vi "Sort 2 Column Array By First Column.vi"(11 "原始座標陣列":cluster{"X":dbl, "Y":dbl}[](array[cluster])=[{"X"=13.0, "Y"=100.0}, {"X"=12.0, "Y"=100.0}, {"X"=11.0, "Y"=100.0}, {"X"=22.0, "Y"=200.0}, {"X"=21.0, "Y"=200.0}, {"X"=24.0, "Y"=200.0}, {"X"=23.0, "Y"=200.0}, {"X"=33.0, "Y"=300.0}, {"X"=31.0, "Y"=300.0}, {"X"=34.0, "Y"=300.0}, {"X"=32.0, "Y"=300.0}, {"X"=35.0, "Y"=300.0}, {"X"=46.0, "Y"=400.0}, {"X"=44.0, "Y"=400.0}, {"X"=45.0, "Y"=400.0}, {"X"=43.0, "Y"=400.0}, {"X"=41.0, "Y"=400.0}, {"X"=42.0, "Y"=400.0}]) -> (3 "已完成排序座標陣列":cluster{"X":dbl, "Y":dbl}[][](array[cluster]))   [LabVIEW 2015]
panel:
  out "座標點數":i32
  out "輸入座標":dbl[][](array[numeric])
  in  "X個數":i32=5
  in  "Y個數":i32=5
  in  "分割閥值":dbl=75.0 format="%#_13g"
  in  "繪出結果?":bool=TRUE
  out "Image":T1(plugin-control)
  out "Array 2":errorcluster[](array[cluster])
  out "處理點數y":i32
  out "第一次排序結果之次要陣列":dbl[](array[numeric])
  out "第一次排序結果之主要陣列":dbl[](array[numeric])
  out "已完成排序陣列":dbl[][][](array[numeric])
  out "以各排數量切割之次要陣列":dbl[][](array[numeric])
  out "各排數量":i32[](array[numeric])
  out "以各排數量切割之主要陣列":dbl[][](array[numeric])
  out "第一次排序結果_X":dbl[](array[numeric])
  out "第一次排序結果_Y":dbl[](array[numeric])
  in  "主排序參考目標":enum16{"X排序", "Y排序"}(ring)
  out "第一次排序結果":dbl[][](array[numeric])
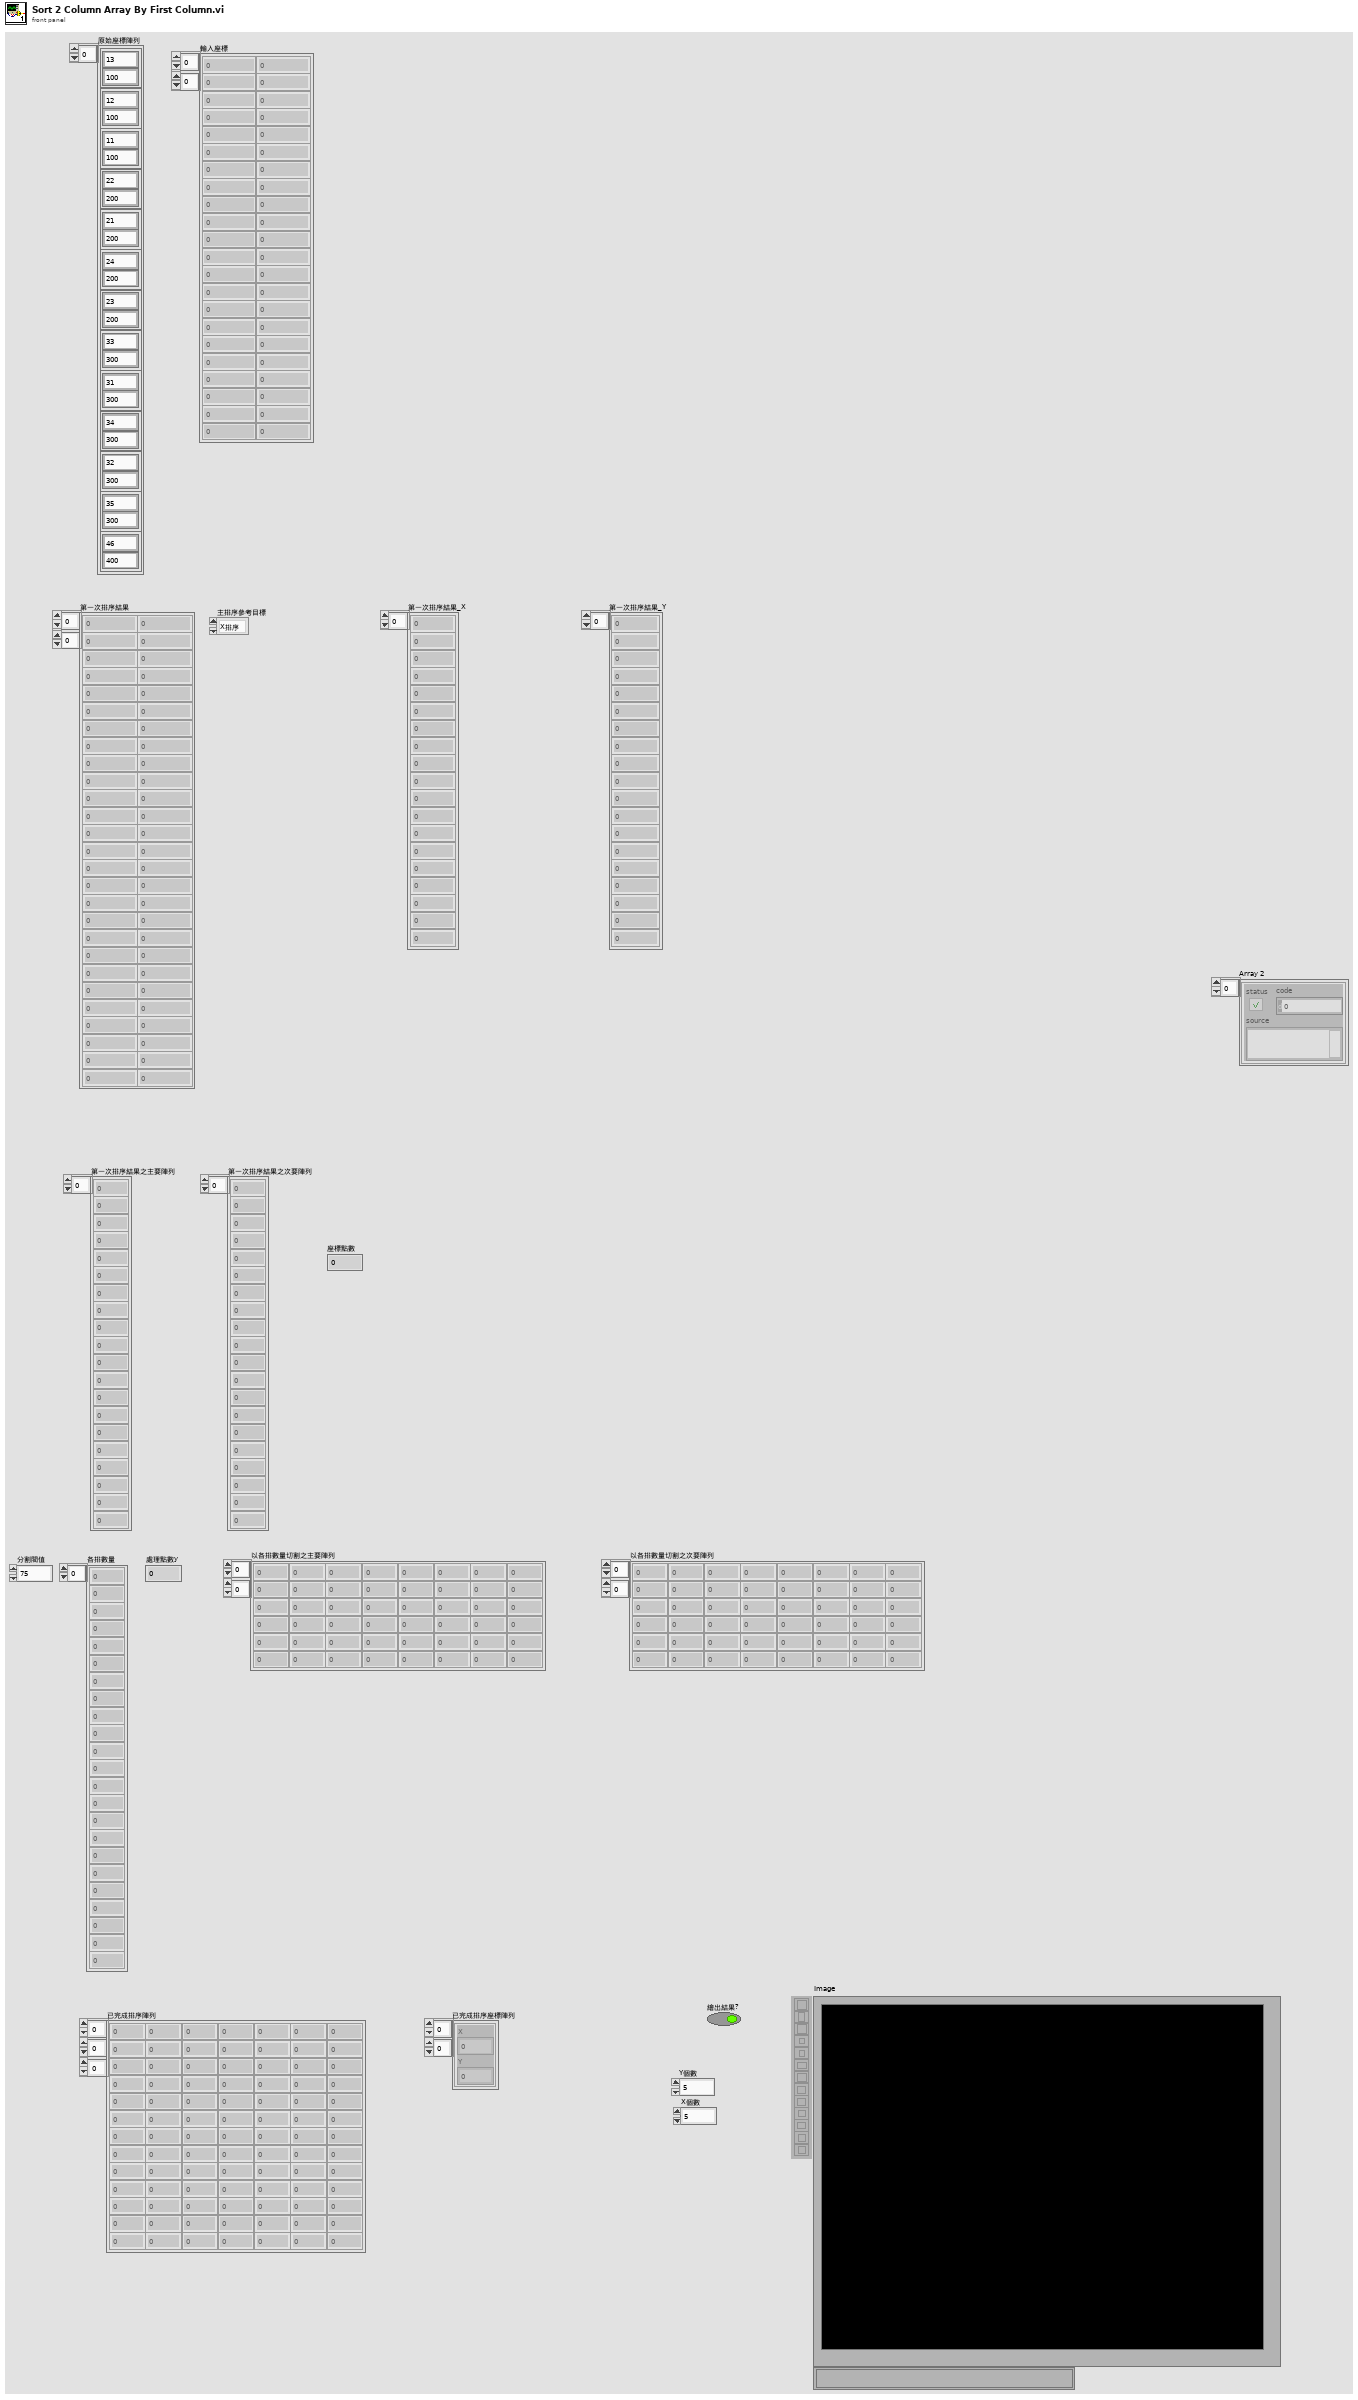
[diagram p1: front panel]
types:
  T1 = typedef "IMAQ Image.ctl" = refnum<image>
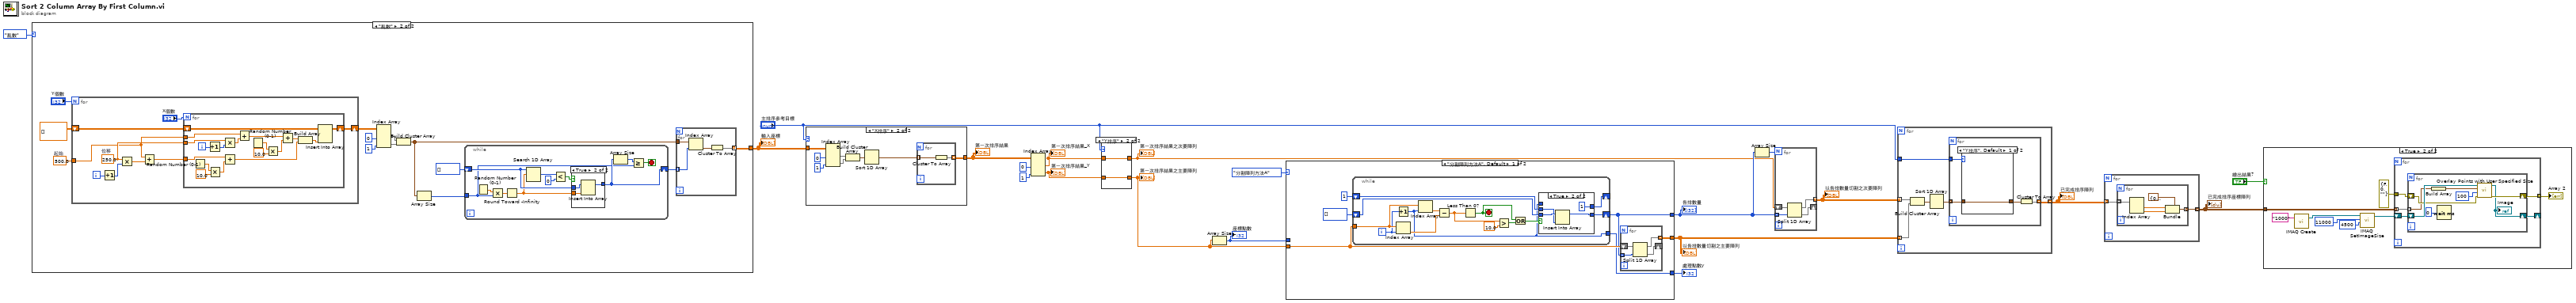
[diagram p0: block diagram]
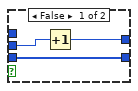
[diagram p2: hidden frame]
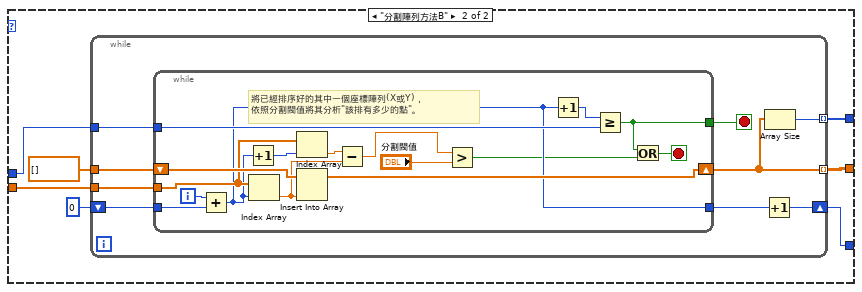
[diagram p3: hidden frame]
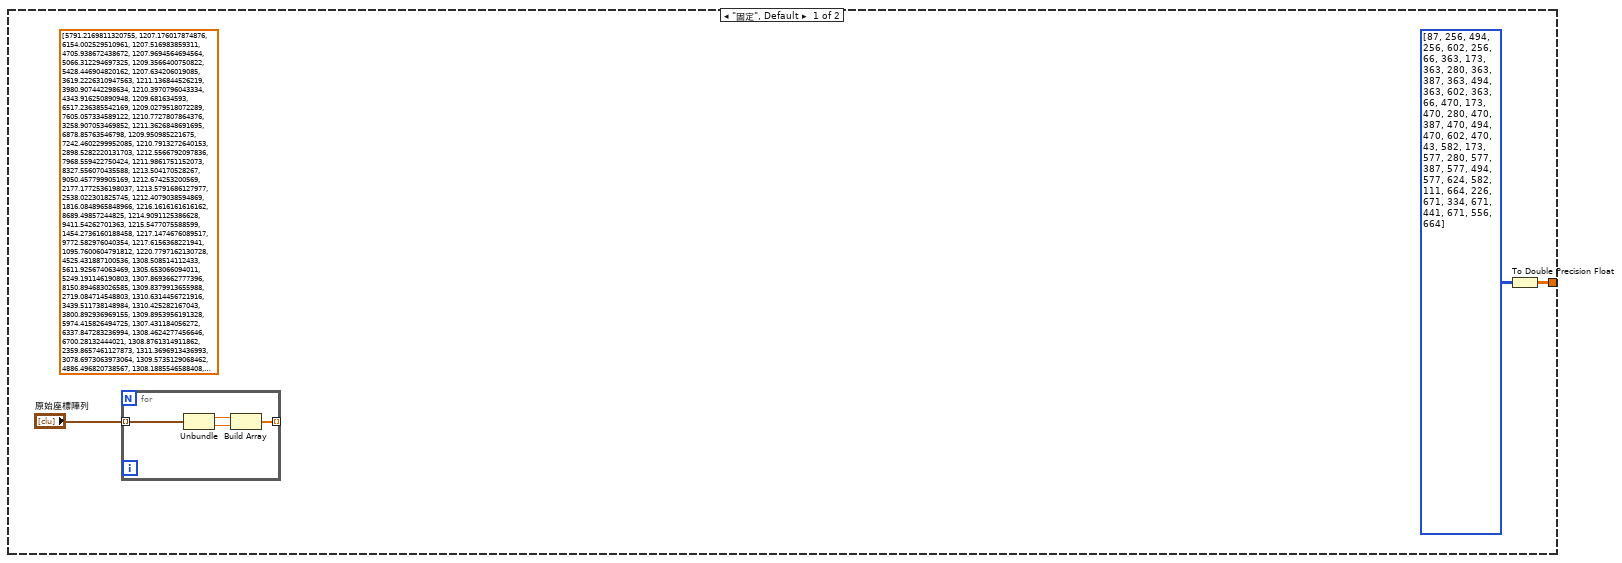
[diagram p4: hidden frame]
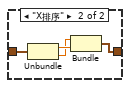
[diagram p7: hidden frame]
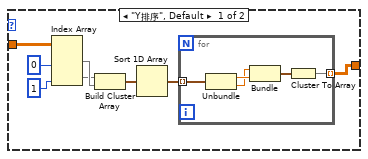
[diagram p9: hidden frame]
diagram:
  n1 = case shown="\"亂數\"" enum16{"固定", "亂數"}."亂數" {
    tunnel: [w21 w32] -> w6
    frame "固定", Default {
      (unwired) dbl[][] [[5791.2169811320755, 1207.176017874876], [6154.002529510961, 1207.516983859311], [4705.938672438672, 1207.9694564694564], [5066.312294697325, 1209.3566400750822], [5428.446904820162, 1207.634206019085], [3619.2226310947563, 1211.136844526219], [3980.907442298634, 1210.3970796043334], [4343.916250890948, 1209.681634593], [6517.236385542169, 1209.0279518072289], [7605.057334589122, 1210.7727807864376], [3258.907053469852, 1211.3626848691695], [6878.85763546798, 1209.950985221675], [7242.4602299952085, 1210.7913272640153], [2898.5282220131703, 1212.5566792097836], [7968.559422750424, 1211.9861751152073], [8327.556070435588, 1213.504170528267], [9050.457799905169, 1212.674253200569], [2177.1772536198037, 1213.5791686127977], [2538.022301825745, 1212.4079038594869], [1816.0848965848966, 1216.1616161616162], [8689.49857244825, 1214.9091125386628], [9411.54262701363, 1215.5477075588599], [1454.2736160188458, 1217.1474676089517], [9772.582976040354, 1217.6156368221941], [1095.7600604791812, 1220.7797162130728], [4525.431887100536, 1308.508514112433], [5611.925674063469, 1305.653066094011], [5249.191146190803, 1307.8693662777396], [8150.894683026585, 1309.8379913655988], [2719.084714548803, 1310.6314456721916], [3439.511738148984, 1310.425282167043], [3800.892936969155, 1309.8953956191328], [5974.415826494725, 1307.431184056272], [6337.847283236994, 1308.4624277456646], [6700.28132444021, 1308.8761314911862], [2359.8657461127873, 1311.3696913436993], [3078.6973063973064, 1309.5735129068462], [4886.496820738567, 1308.1885546588408], [7062.827751196172, 1309.4813397129187], [7427.45506669787, 1309.2068804118885], [8511.356658376668, 1311.258421885598], [8872.234061930783, 1311.655510018215], [4162.5688587086015, 1309.666428401239], [7788.041149425288, 1310.5857471264367], [1635.5710637352877, 1313.0397512769264], [1997.7501715069745, 1312.5035444774753], [9232.897453387903, 1313.3672123692588], [1274.6067873303168, 1317.8484162895927], [9593.201644660643, 1315.2645355570999], [9952.616504854368, 1317.176499875529], [5430.564612326044, 1403.6607852882703], [5793.774098695985, 1404.0516491945793], [6155.000251130085, 1403.7762430939226], [6518.11789807364, 1405.2377468910022], [4344.622950819672, 1406.5009643201543], [3619.45225714961, 1408.1621366107304], [7245.313248594475, 1408.0041554632119], [3258.734342012667, 1409.54890921886], [4707.38623046875, 1409.024169921875], [5068.421871049305, 1406.161567635904], [6882.053212358999, 1407.822216772928], [7608.443792155883, 1407.1306520109918], [2179.6376459143967, 1409.6850680933853], [3980.357344632768, 1409.775188323917], [7969.418336292163, 1407.645447628709], [8331.37233032748, 1408.6473659231135], [8692.269665567594, 1409.7538860103627], [2897.7616095307562, 1408.684172137126], [9053.6467124632, 1408.6459764474976], [2539.6725509696666, 1410.0730979612133], [1099.072462077013, 1414.2942823803967], [1817.3156834873253, 1413.0348258706467], [9414.970602828082, 1413.0022326966014], [9773.850379251284, 1414.3944213359432], [1455.220919100048, 1414.8228817616084], [5612.357605177994, 1502.180690399137], [4526.020811654526, 1502.9622788761706], [5247.853276353277, 1502.6335146335146], [5974.880021715527, 1502.6471226927254], [7788.572317880795, 1503.4405298013246], [8873.339039345938, 1505.144098109351], [6335.7773246329525, 1503.1606851549755], [4162.258917278016, 1506.8547938274728], [4886.88221614227, 1504.3124487004104], [6699.960096411355, 1503.6459560792716], [7065.031008783604, 1504.9840298110194], [7427.821718627194, 1505.8352108986114], [8150.256849315068, 1507.4307729941293], [8512.864804745428, 1508.1668314384578], [3800.291616477957, 1510.511443025777], [2359.2007088474666, 1507.0719348910475], [3077.414345769837, 1506.1037834997373], [3438.0564182194616, 1505.6392339544514], [9234.197371844914, 1507.5016913869372], [2716.955280172414, 1506.9234913793102], [1277.1903353057198, 1513.2260848126232], [1636.1105111591073, 1511.6306695464364], [1996.1912561258705, 1510.1307712148568], [9595.101593625497, 1512.0701195219124], [9952.666338305657, 1514.8809456797073], [6516.624943617501, 1607.9104645917907], [3616.434411500449, 1609.2830188679245], [3255.1358316452847, 1611.067521944632], [5066.782830573827, 1609.6119301428896], [6154.794930875576, 1608.5082949308755], [2895.820072743805, 1611.7272107297113], [4342.289616252821, 1610.3690744920993], [4705.4812142038945, 1610.4215349369988], [5427.558903488899, 1610.066606252832], [3978.4939475453934, 1610.3730105357542], [5790.527250608273, 1608.66399026764], [7242.933211344922, 1610.0388838060385], [7968.398886827458, 1610.7219387755101], [8691.733163028333, 1611.2183000464468], [9051.415883668904, 1612.092841163311], [6879.367298578199, 1610.8947867298577], [7605.550802779775, 1610.9796309609394], [9772.936148874527, 1614.2090483619345], [2537.1703652334722, 1613.1026352288488], [8329.660801564027, 1611.8164711632453], [9413.658141612686, 1613.2977440250168], [2174.5085707667363, 1615.4067639564512], [1454.8072275676884, 1620.3620496755427], [1098.2838932570885, 1618.710507505361], [1813.765814112811, 1619.6268554464489], [3432.7249308871574, 1714.0794169389294], [3795.35187044941, 1715.1995982927442], [4156.692948090108, 1716.0034280117532], [3073.052139379964, 1716.205995388163], [1632.0854131330263, 1718.6629512963411], [6330.915481832543, 1712.7777777777778], [8872.46767411301, 1717.6349540078843], [2714.7747580044675, 1716.6056093323405], [5969.166583229036, 1713.5344180225281], [6694.592108735814, 1714.9918184217472], [8508.792178917081, 1715.5417211613915], [1989.1021611001966, 1719.932956777996], [2353.5285641418004, 1719.878857434328], [5606.145459209852, 1716.39763981529], [7058.01411136537, 1715.0333079074499], [7421.791013584117, 1715.689132706374], [4519.88543328017, 1716.199893673578], [5243.284035133041, 1717.7452854559544], [7783.365578231293, 1717.2462585034014], [9232.259290072103, 1719.4728230726566], [1272.845079285175, 1720.5801661213188], [4882.937808219178, 1715.6323287671232], [8144.936657681941, 1717.1366576819407], [9591.000678426051, 1722.3915875169607], [9949.065279868619, 1723.254139865882], [4704.614984155726, 1811.9834766862834], [5786.604245164532, 1809.6865109269029], [6514.535163776493, 1813.2603564547205], [6877.67354965585, 1811.9594395280235], [6151.978198370867, 1813.089602299952], [3978.3221362977283, 1814.329386176897], [7240.83000997009, 1812.3277666999004], [7965.428588897041, 1815.9814135485449], [2534.981555834379, 1816.826850690088], [3615.618245699055, 1813.1737339471772], [4341.0246138996135, 1814.5381274131273], [5426.583291010666, 1811.312341289995], [8328.642644135189, 1815.0099403578529], [9052.143729743206, 1816.426576913488], [1815.0420583273078, 1819.9110629067245], [2895.753032928943, 1813.921020054469], [3253.824297438448, 1815.028848545138], [5065.478394303953, 1813.887061134299], [9414.352200457899, 1817.40422284406], [1098.6733201091, 1819.5578973468882], [2173.020701412567, 1819.3468095470043], [7603.653050672182, 1814.8753877973113], [1454.524729891957, 1821.038175270108], [8690.614173228347, 1814.9613681102362], [9773.988752556237, 1818.053680981595], [5247.1742229492875, 1908.279738256602], [5610.254849263847, 1908.1423229726572], [5972.489056087551, 1909.0362517099863], [6334.6076212471135, 1908.3951501154734], [7059.915295480881, 1908.824333719583], [7423.796435272045, 1910.078330206379], [7785.741147882434, 1910.896551724138], [4159.929595375723, 1910.3260115606936], [3437.6755601755603, 1913.949641949642], [4885.988111888112, 1910.7888111888112], [6696.816946348381, 1909.472465138265], [8148.402939804013, 1912.7727484834345], [2356.2925696594425, 1913.7811383662777], [2716.1378404204493, 1914.0993788819876], [3077.4003200731595, 1915.6213991769548], [3798.951251489869, 1912.8746126340882], [4523.41652344709, 1912.9629265897372], [9235.39332096475, 1913.7284322820037], [8509.45624256837, 1914.235196195006], [8873.527777777777, 1913.6053639846743], [9596.565009560229, 1914.8814531548758], [1636.0460588793921, 1919.2863247863247], [1996.2744091668656, 1918.7428980663642], [1279.4822637106183, 1920.5913652275378], [9952.766458852868, 1918.4258104738155], [6153.8170227429355, 2009.859637031932], [5066.484104721832, 2009.921458625526], [5789.492005643076, 2009.0002351281448], [5430.319796353303, 2008.9040966137816], [6517.169457067687, 2010.6376464960535], [6880.849392165691, 2012.3572714993247], [9055.709640745794, 2013.1377899045021], [3258.352574653186, 2014.5713613919586], [4705.719306466729, 2012.4835988753514], [7243.692893401016, 2011.9864636209813], [7607.454435288415, 2010.9663111972854], [7968.672670230072, 2012.3434812921219], [2897.9132035146044, 2014.5832343861316], [4343.976258649487, 2012.3120973514674], [8330.214816535068, 2013.349280074315], [3620.0517077798863, 2014.5493358633776], [3982.5302308974055, 2014.098309926208], [8693.775339002528, 2013.7924615031027], [2538.751615992339, 2015.047402441944], [9415.60828182942, 2015.435846724351], [2177.8562231759656, 2016.5591320934668], [9778.519986216403, 2018.1157822191592], [1817.681731909846, 2020.0873072360616], [1457.2464114832535, 2021.4196172248803], [1101.999758337361, 2022.1652972450458], [5248.732352237377, 2107.517827231395], [5973.682421227198, 2108.479270315091], [6700.691815856778, 2109.379446640316], [5612.669209105844, 2111.2762262379724], [7425.028975428836, 2110.2329624478443], [4887.984679665738, 2112.0299442896935], [6335.250118315192, 2111.0795078088026], [7788.795105566219, 2112.734404990403], [8150.576462459696, 2112.7206356517736], [8513.043503890593, 2111.8389530771046], [3801.8130515559683, 2113.5673478866697], [4525.211808809747, 2112.285613870665], [9235.167302192564, 2114.0865109628216], [2360.203281027104, 2115.401569186876], [2719.848698352042, 2113.9842369238117], [3079.9432965484857, 2113.6583705095095], [3440.210061884025, 2113.863167545267], [7062.920090239848, 2113.2161006886727], [4164.457772621809, 2114.2498839907194], [8875.46652922629, 2112.535774921174], [1998.6349448486271, 2115.715090354377], [9598.689484126984, 2117.3263888888887], [9954.744780152298, 2119.186809137804], [1639.7413207089098, 2120.402767662054], [1279.489117577478, 2121.8142890939203], [5431.053639360893, 2207.2916560994167], [6519.0869934481925, 2208.044892016501], [5792.554679802955, 2208.185960591133], [6154.561583577713, 2207.697458455523], [2899.03954050786, 2211.010882708585], [4707.999880753637, 2210.989983305509], [5068.351178781925, 2209.5230844793714], [6880.464836832785, 2209.094105742474], [7607.18498890806, 2209.4397337934433], [7969.78310727497, 2210.7551171393343], [3260.349441476445, 2212.7042253521126], [7244.3662109375, 2211.40087890625], [8331.217961405246, 2210.521276595745], [3623.0323997151672, 2213.4051744600047], [8694.145669291338, 2212.9379921259842], [3983.87895256917, 2211.9426877470355], [4344.828294280675, 2211.371126228269], [2540.2300098716682, 2214.078232971372], [9053.753157894736, 2212.271052631579], [2180.4587576374747, 2213.516547861507], [9414.56498194946, 2214.3120165033524], [1457.543881033642, 2217.4256460263286], [1820.8730694980695, 2219.265926640927], [9778.070615623383, 2216.237454733575], [1101.8869002284844, 2223.269611576542], [3441.5759493670885, 2307.637921940928], [5612.339923643305, 2305.1298063812383], [7062.993651204975, 2308.5752785695777], [4887.433227344992, 2306.98675145734], [5973.299479166667, 2306.385677083333], [6337.661087339542, 2308.794613642084], [4164.20913526701, 2307.685551640011], [4524.341320553781, 2305.896432374867], [5250.014176663031, 2305.5981461286806], [6700.81314699793, 2308.371376811594], [7425.287467362924, 2308.0046997389036], [7787.878064856314, 2308.0487740574745], [2719.438112429087, 2310.4272821041773], [3080.6123244929795, 2309.9682787311494], [3801.5416103755742, 2307.9921642799245], [8150.205319148936, 2309.8574468085108], [2362.5581613508443, 2310.08818011257], [8512.328911748782, 2308.986193827829], [2001.6717537506468, 2314.1324366270046], [8873.817425083242, 2310.0826859045505], [9234.317637452368, 2311.2874251497005], [9597.190749863164, 2313.4395183360703], [9954.403873140613, 2316.639489194499], [1639.6540974680097, 2315.3972229784918], [1279.6960380756368, 2320.3174684846927], [8330.202048007048, 2413.715481171548], [1096.627214902317, 2421.915720127215], [5793.369089316988, 2413.4614711033273], [6156.94052464948, 2411.7476255088195], [3981.7318511796734, 2415.4820780399273], [5068.8699074074075, 2412.4949074074075], [5431.829401290897, 2413.719563765858], [7243.78610919143, 2412.134761575674], [7605.668177697189, 2413.038984587489], [7967.357369975017, 2413.8964342493755], [4345.859130231471, 2413.3362169745146], [4707.703206141341, 2414.1840144502144], [6518.28573104905, 2412.7146209809903], [6880.357748469148, 2413.0977390485164], [3622.2240517828754, 2414.682262094027], [8691.513750592698, 2415.5320056899004], [2538.295429083576, 2417.556800358503], [2900.3592007434945, 2415.75906133829], [3261.9175365344468, 2416.071213175597], [9051.614809454897, 2415.5800771828267], [9412.444, 2418.5181176470587], [2180.4168634860653, 2419.272319319792], [9774.410749506904, 2419.995315581854], [1458.014869888476, 2422.5450743494425], [1820.7853434033514, 2422.048855322162], [7423.036790123457, 2516.8414814814814], [4887.03853706431, 2517.189003436426], [6698.659789947487, 2514.7274318579643], [3080.121237659523, 2518.5157717312786], [5612.117874736101, 2515.69716162327], [5974.3404593207915, 2515.898851698021], [3441.0567257060793, 2519.2307324078506], [5249.530179640718, 2516.226107784431], [7061.295358123284, 2518.5133516346395], [2718.0598626104024, 2521.786064769382], [2001.6912596401028, 2522.4413881748073], [3802.4208139249818, 2519.1600882569255], [6337.084878401156, 2519.3845412954493], [8870.51100671141, 2520.389798657718], [4164.208527131783, 2517.4346253229974], [7786.674478527608, 2518.0191411042947], [4524.88011988012, 2519.7874625374625], [8509.584243369734, 2520.521840873635], [1639.5500495540139, 2523.1402378592666], [8147.402301790281, 2521.40358056266], [1277.4132397191574, 2528.26705115346], [2359.226819541376, 2523.3158025922235], [9592.892588753562, 2522.689038611039], [9230.387912087912, 2523.200824175824], [9952.249753208293, 2527.0788323226625], [5070.825005892058, 2615.7834079660615], [5431.699376947041, 2615.5398993529834], [6156.222182680902, 2615.0688018979836], [6518.488146040778, 2616.7491702228544], [6881.878078223081, 2616.4167069048767], [2902.763772175537, 2617.2766106442577], [3983.8963698798134, 2615.8180034338975], [5796.037472714043, 2615.085132185302], [2540.185934489403, 2618.995183044316], [3623.964962121212, 2616.5991950757575], [7607.497571046879, 2616.1141607966965], [3263.299901671583, 2618.1482300884954], [4348.266404199475, 2617.0372226198997], [4708.2179866765355, 2617.26745620528], [7243.497597308986, 2617.371696299856], [7969.716850167544, 2618.648157012925], [1822.5514257860102, 2620.26102851572], [2181.9689182574643, 2620.559716103769], [8330.935110786462, 2620.747017287558], [8693.1137487636, 2619.8081107814046], [1459.1380733944954, 2625.107339449541], [9052.026473526474, 2619.4125874125875], [9412.43154158215, 2622.208164300203], [9774.795795070082, 2623.6872885451908], [1098.5962264150944, 2626.583254716981], [4530.49663623258, 2712.9591542527633], [5255.509969143129, 2713.6907192024687], [5617.3297378798425, 2714.568081651589], [5981.173020856694, 2716.2996187485983], [6702.9324074074075, 2713.706712962963], [4167.960863541907, 2714.8540752712997], [4892.438146811071, 2713.677015643803], [7067.205800464038, 2715.991879350348], [3447.269899359561, 2716.0983531564502], [6341.353219927096, 2714.8162818955043], [7428.671260732038, 2716.3145051965657], [2724.7040769052583, 2718.662728746815], [3807.6274158911956, 2714.9398711524695], [7789.469696969697, 2716.6572543618], [8151.380858924036, 2716.364350034634], [8515.167982354307, 2717.946134200139], [2005.4705332086062, 2720.3550046772684], [2363.1271817547126, 2718.6167093320923], [3085.409580698056, 2718.480440384165], [8874.301165331392, 2718.652100024278], [1279.4872175302442, 2722.9680438256105], [1643.7951861943689, 2721.7824704813806], [9235.233830845771, 2720.355721393035], [9594.670708283313, 2721.6216086434574], [9953.702181097158, 2724.681031064111], [4351.532228778938, 2814.7793917385384], [4713.017429938483, 2813.574618364092], [5075.223098330242, 2813.2590445269016], [5438.657355679702, 2814.4511173184355], [6161.42585812357, 2814.179633867277], [5800.098030438675, 2816.199418084154], [6524.636524404622, 2814.4024994105166], [7248.455440900563, 2815.4953095684805], [7611.352062588905, 2814.5599810336653], [3988.994145199063, 2815.509836065574], [6885.94406531806, 2813.558859371192], [3628.177997671711, 2816.1844004656577], [8334.506838009904, 2818.269511907569], [7972.427917351491, 2818.228926978164], [2546.072148419606, 2820.1408612001833], [3268.46, 2818.753563218391], [2907.402585410896, 2819.4434441366575], [1826.7451956471405, 2822.9694373697616], [2186.9701925307354, 2821.5884945488287], [8695.439464493596, 2820.207217694994], [1461.4986184664979, 2824.1853557448767], [9055.015810776626, 2821.408044523147], [9415.225345167653, 2821.7058678500985], [1101.4419369471536, 2826.7026536629623], [9776.254446640316, 2823.951333992095], [6344.134682892582, 2913.471331617131], [5982.747816091954, 2913.9094252873565], [7431.626306013466, 2915.108195960065], [4172.039186393932, 2914.48793380832], [4533.994316915534, 2914.401604635614], [7068.6510895883775, 2913.9970944309925], [3449.376069364162, 2915.7581502890175], [4896.845881310895, 2915.4676705048714], [5259.05535265921, 2914.779045879936], [5620.630761994355, 2915.3029162746943], [6705.708517570398, 2914.466604607866], [8153.402667290594, 2917.1017781937294], [7793.676442984514, 2917.017832003754], [3809.8314020857474, 2916.4486674391655], [2006.4374714742128, 2921.897307165678], [8515.554447312838, 2919.702651959634], [8876.092145015105, 2919.896351382756], [2727.491670522906, 2920.660573808422], [3087.8775605214155, 2920.6317504655494], [1645.2203214695753, 2922.740528128588], [2366.529809035864, 2922.4219841639497], [9236.410976226605, 2921.716995447648], [9595.018650996422, 2922.309402146142], [1282.4443538998835, 2925.2696158323633], [9951.857612960384, 2924.2308568535627], [3990.39806763285, 3014.1821256038647], [4715.53953147877, 3012.4882869692533], [5801.062022900764, 3012.28125], [4353.162387066096, 3013.452924393723], [6163.387980173482, 3012.0468401486987], [6526.057816377172, 3012.3640198511166], [5440.239277108434, 3013.449879518072], [7249.366066966517, 3011.039980009995], [5077.724840451645, 3012.7844869906726], [6886.821946169773, 3011.266304347826], [7610.535495716034, 3007.5538555691555], [3267.6351482741857, 3017.0165289256197], [3629.666626301768, 3016.3993703075807], [7975.841638981174, 3012.4731450719823], [8334.069898534386, 3012.9512401352877], [2906.407448107448, 3017.792673992674], [8694.568808567603, 3013.641231593039], [1826.6714147754708, 3020.2863351038145], [2545.520343908937, 3019.1266650520706], [9055.34398976982, 3016.8831202046035], [2186.167820925056, 3019.4546129112045], [9415.903714832013, 3019.235454793772], [1462.7366849773107, 3023.5345115834725], [1100.8095998035847, 3025.130861772649], [9774.860292199322, 3021.8236368379858], [4172.46048024012, 3112.396948474237], [4536.090310559006, 3111.7875776397514], [5619.468373090324, 3108.8209595282765], [4896.098458676588, 3108.4562848790856], [5258.901501423764, 3109.792907067046], [5982.520722635494, 3109.4766206163654], [3448.2495476867407, 3113.6634789351256], [6343.703609701071, 3108.322617033277], [3810.3542836221627, 3113.7759336099584], [6703.1737044145875, 3106.7287268074215], [3087.8186983471073, 3115.925361570248], [2368.09423172551, 3118.2555942317254], [2725.8445945945946, 3116.163981288981], [1282.6567398119123, 3121.246342737722], [2006.4220879403445, 3118.6150681409104], [9235.67416378316, 3113.6372549019607], [1644.0447705041383, 3118.826435916729], [9594.389253486464, 3118.299425758819], [9951.107698900158, 3118.59977146122], [1819.9716391246093, 3219.8128628852164], [4350.037811178957, 3213.739314232034], [5435.479185938945, 3215.4761794634596], [5796.171014492754, 3214.79154589372], [4712.182858477347, 3214.232134516581], [5073.849610757254, 3214.2297711724464], [6158.311000269615, 3217.6047452143434], [3624.863824408182, 3216.9866697310963], [3987.4235757295046, 3215.4678091709125], [3263.149474689589, 3218.2184813753584], [2541.306586270872, 3220.746521335807], [2901.4476145930776, 3220.966557530402], [2180.899198302287, 3222.378684272577], [1455.9328180737218, 3225.8121284185495], [7963.47076372315, 3226.7488066825777], [1094.2902325581395, 3227.923023255814], [8690.688751406075, 3237.755905511811], [9763.40395480226, 3229.8458882611426], [7603.004116529449, 3228.0060164661177], [8326.659253945481, 3231.2611190817793], [6518.36497461929, 3226.594923857868], [7242.8767780350645, 3227.8511412504135], [9048.118569636135, 3230.7565872020077], [6879.875815870835, 3226.727241497767], [9404.376605915746, 3232.993725724529], [3442.5009789525207, 3320.513215859031], [4887.796898830707, 3315.9313675648195], [8505.319880239522, 3321.9978443113773], [3802.511938023876, 3316.48158496317], [8144.35543667579, 3320.8579248569295], [2358.84423863363, 3320.9109935049314], [2720.1936470588234, 3324.041411764706], [5611.086652871185, 3319.5186239006725], [8866.114169215087, 3322.6929153924566], [6335.574074074074, 3318.654857756307], [6696.924495289368, 3317.980619111709], [7783.136226415094, 3320.640251572327], [3080.6293714844705, 3322.435069699193], [7060.406190862395, 3318.021897810219], [5250.042534504391, 3320.8948557089084], [5974.941399112503, 3318.861654920386], [1999.0048155978388, 3326.293399107353], [4165.41658084449, 3320.419412976313], [7423.605372978613, 3320.4358372456963], [4526.90813093981, 3318.81626187962], [9224.642290249432, 3323.5246598639455], [9583.969532100109, 3324.041077257889], [9944.384848484848, 3325.6742424242425], [1636.9337623012868, 3327.442846328539], [1274.110775427996, 3329.471550855992]] ("Array")
      n2 = for {
        tunnel: "原始座標陣列" -> [w27] mode=indexing
        tunnel: [w24] -> _ mode=indexing
        n3 = Unbundle(w27) -> ("X"=w26:dbl, "Y"=w25:dbl)
        n4 = Build Array(w26, w25) -> (w24:dbl[])
      }
      n5 = To Double Precision Float(number=i32[][] [[87, 256], [494, 256], [602, 256], [66, 363], [173, 363], [280, 363], [387, 363], [494, 363], [602, 363], [66, 470], [173, 470], [280, 470], [387, 470], [494, 470], [602, 470], [43, 582], [173, 577], [280, 577], [387, 577], [494, 577], [624, 582], [111, 664], [226, 671], [334, 671], [441, 671], [556, 664]] ("array")) -> (double precision float=w21:dbl[][])
    }
    frame "亂數" {
      w31 = 500.0  # 起始
      n6 = for {
        N: "Y個數" -> [_]
        shift-right: [w65] -> w34
        shift-left: dbl[][] [] -> [w66]
        tunnel: w31 -> [w60]
        i -> [w68]
        w61 = 250.0  # 位移
        n7 = Increment(x=w68) -> (x+1=w67:i32)
        n8 = Multiply(x=w61, y=w67) -> (x*y=w63:dbl)
        n9 = Add(x=w60, y=w63) -> (x+y=w62:dbl)
        n10 = for {
          N: "X個數" -> [_]
          shift-right: [w85] -> w65
          shift-left: w66 -> [w86]
          tunnel: w62 -> [w71]
          tunnel: w60 -> [w82]
          tunnel: w61 -> [w79]
          i -> [w84]
          n11 = Random Number (0-1)() -> (number: 0 to 1=w75:dbl)
          n12 = Increment(x=w84) -> (x+1=w81:i32)
          n13 = Multiply(x=w75, y=10.0) -> (x*y=w73:dbl)
          n14 = Multiply(x=w79, y=w81) -> (x*y=w80:dbl)
          n15 = Add(x=w71, y=w73) -> (x+y=w70:dbl)
          n16 = Add(x=w82, y=w80) -> (x+y=w72:dbl)
          n17 = Random Number (0-1)() -> (number: 0 to 1=w78:dbl)
          n18 = Multiply(x=w78, y=10.0) -> (x*y=w76:dbl)
          n19 = Add(x=w72, y=w76) -> (x+y=w69:dbl)
          n20 = Build Array(w69, w70) -> (w83:dbl[])
          n21 = Insert Into Array(array=w86, new element=w83) -> (w85:dbl[][])  [unwired: 2 in]
        }
      }
      n22 = Index Array(array=w34, index (col) #1=0 ("disabled index (col)"), index (col) #2=1 ("index (col)")) -> (element #1=w35:dbl[], element #2=w36:dbl[])  [unwired: 2 in]
      n23 = Build Cluster Array(w35, w36) -> (w33:cluster{"Y":dbl, "Y":dbl}[])
      n24 = Array Size(array=w33) -> (size(s)=w29:i32)
      n25 = while {
        tunnel: w29 -> [w43]
        shift-right: [w44] -> w28
        shift-left: i32[] [] -> [w50]
        stop <- w45 stop-if-true
        n26 = Random Number (0-1)() -> (number: 0 to 1=w51:dbl)
        n27 = Multiply(x=w51, y=w43) -> (x*y=w42:dbl)
        n28 = Round Toward -Infinity(1:w42) -> (0:w41:dbl)
        n29 = Search 1D Array(1D array=w50, element=w41) -> (index of element=w47:i32)  [unwired: 1 in]
        n30 = Less?(x=w47, y=0) -> (x < y?=w48:bool)
        n31 = case shown="True" w48 {
          tunnel: w50 -> [w52 w55]
          tunnel: w41 -> [_ w53]
          tunnel: [w52 w54] -> w44
          frame False {
          }
          frame True {
            n32 = Insert Into Array(array=w55, new element=w53) -> (w54:i32[])  [unwired: 1 in]
          }
        }
        n33 = Array Size(array=w44) -> (size(s)=w46:i32)
        n34 = Greater Or Equal?(x=w46, y=w43) -> (x >= y?=w45:bool)
      }
      n35 = for {
        tunnel: w33 -> [w59]
        tunnel: [w57] -> w32 mode=indexing
        tunnel: w28 -> [w56] mode=indexing
        n36 = Index Array(array=w59, index=w56) -> (element=w58:cluster{"Y":dbl, "Y":dbl})
        n37 = Cluster To Array(cluster=w58) -> (array=w57:dbl[])
      }
    }
  }
  "輸入座標" <- w6
  n38 = case shown="\"X排序\"" "主排序參考目標" {
    tunnel: w6 -> [w89 w104]
    tunnel: [w91 w102] -> w18
    frame "Y排序", Default {
      n39 = Index Array(array=w89, index (col) #1=0 ("index (row)"), index (col) #2=1 ("index (col)")) -> (element #1=w94:dbl[], element #2=w87:dbl[])  [unwired: 2 in]
      n40 = Build Cluster Array ("Index & Bundle Cluster Array")(w87, w94) -> (w93:cluster{"Y":dbl, "Y":dbl}[])
      n41 = Sort 1D Array(array=w93) -> (sorted array=w92:cluster{"Y":dbl, "Y":dbl}[])
      n42 = for {
        tunnel: w92 -> [w98] mode=indexing
        tunnel: [w99] -> w91 mode=indexing
        n43 = Unbundle(w98) -> ("Y"=w97:dbl, "Y"=w96:dbl)
        n44 = Bundle("Y"=w96, "Y"=w97) -> (w95:cluster{"Y":dbl, "Y":dbl})  [unwired: 1 in]
        n45 = Cluster To Array(cluster=w95) -> (array=w99:dbl[])
      }
    }
    frame "X排序" {
      n46 = Index Array(array=w104, index (col) #1=0 ("disabled index (col)"), index (col) #2=1 ("index (col)")) -> (element #1=w107:dbl[], element #2=w103:dbl[])  [unwired: 2 in]
      n47 = Build Cluster Array(w107, w103) -> (w106:cluster{"Y":dbl, "Y":dbl}[])
      n48 = Sort 1D Array(array=w106) -> (sorted array=w105:cluster{"Y":dbl, "Y":dbl}[])
      n49 = for {
        tunnel: w105 -> [w109] mode=indexing
        tunnel: [w108] -> w102 mode=indexing
        n50 = Cluster To Array(cluster=w109) -> (array=w108:dbl[])
      }
    }
  }
  "第一次排序結果" <- w18
  n51 = Index Array(array=w18, index (col) #1=0 ("disabled index (col)"), index (col) #2=1 ("index (col)")) -> (element #1=w17:dbl[], element #2=w16:dbl[])  [unwired: 2 in]
  "第一次排序結果_Y" <- w16
  "第一次排序結果_X" <- w17
  n52 = case shown="\"Y排序\"" "主排序參考目標" {
    tunnel: w17 -> [w111 w112]
    tunnel: w16 -> [w110 w113]
    tunnel: [w111 w113] -> w3
    tunnel: [w110 w112] -> w12
    frame "X排序", Default {
    }
    frame "Y排序" {
    }
  }
  "第一次排序結果之主要陣列" <- w3
  "第一次排序結果之次要陣列" <- w12
  n53 = Array Size(array=w3) -> (size(s)=w4:i32)
  "座標點數" <- w4
  n54 = case shown="\"分割陣列方法A\", Default" enum16{"分割陣列方法A", "分割陣列方法B"}."分割陣列方法A" {
    tunnel: [w115 w150] -> w13
    tunnel: [w114 w148] -> w8
    tunnel: w4 -> [_ w147]
    tunnel: w3 -> [w116 w146]
    tunnel: [w117 w145] -> w2
    frame "分割陣列方法A", Default {
      n55 = while {
        tunnel: w116 -> [w137]
        shift-right: [w131] -> w115
        shift-left: i32[] [] -> [w133]
        shift-right: [w129] -> _
        shift-left: 1 -> [w130]
        tunnel: [w125] -> w114
        i -> [w132]
        stop <- w126 stop-if-true
        n56 = Increment(x=w132) -> (x+1=w125:i32)
        n57 = Index Array(array=w137, index=w132) -> (element=w135:dbl)
        n58 = Index Array(array=w137, index=w125) -> (element=w136:dbl)
        n59 = Subtract(x=w136, y=w135) -> (x-y=w124:dbl)
        n60 = Less Than 0?(x=w124) -> (x < 0?=w126:bool)
        n61 = Greater?(x=w124, y=10.0) -> (0:w128:bool)
        n62 = Or(x=w126, y=w128) -> (x .or. y?=w127:bool)
        n63 = case shown="True" w127 {
          tunnel: w133 -> [w140 w144]
          tunnel: w125 -> [_ _]
          tunnel: [w140 w143] -> w131
          tunnel: w130 -> [w139 w141]
          tunnel: [w138 1] -> w129
          frame False {
            n64 = Increment(x=w139) -> (x+1=w138:i32)
          }
          frame True {
            n65 = Insert Into Array(array=w144, new element=w141) -> (w143:i32[])  [unwired: 1 in]
          }
        }
      }
      n66 = for {
        tunnel: w115 -> [w120] mode=indexing
        tunnel: [w122] -> w117 mode=indexing
        shift-right: [w121] -> _
        shift-left: w116 -> [w123]
        n67 = Split 1D Array(array=w123, index=w120) -> (first subarray=w122:dbl[], second subarray=w121:dbl[])
      }
    }
    frame "分割陣列方法B" {
      n68 = while {
        tunnel: w146 -> [w160]
        tunnel: [w159] -> w145 mode=indexing
        tunnel: [w157] -> w150 mode=indexing
        tunnel: dbl[] [] -> [w158]
        tunnel: w147 -> [w156]
        shift-right: [w152] -> w148
        shift-left: 0 -> [w154]
        stop <- w155 stop-if-true
        n69 = while {
          tunnel: w160 -> [w174]
          shift-right: [w175] -> w159
          shift-left: w158 -> [w176]
          tunnel: w156 -> [w169]
          tunnel: [w166] -> w155
          tunnel: [w164] -> w153
          tunnel: w154 -> [w165]
          i -> [w172]
          stop <- w167 stop-if-true
          # "將已經排序好的其中一個座標陣列(X或Y)，\n依照分割閥值將其分析\"該排有多少的點\"。"
          n70 = Add(x=w172, y=w165) -> (x+y=w164:i32)
          n71 = Increment(x=w164) -> (x+1=w173:i32)
          n72 = Index Array(array=w174, index=w164) -> (element=w170:dbl)
          n73 = Index Array(array=w174, index=w173) -> (element=w171:dbl)
          n74 = Insert Into Array(array=w176, new element=w170) -> (w175:dbl[])  [unwired: 1 in]
          n75 = Subtract(x=w171, y=w170) -> (x-y=w163:dbl)
          n76 = Greater?(x=w163, y="分割閥值") -> (0:w161:bool)
          n77 = Increment(x=w164) -> (x+1=w168:i32)
          n78 = Greater Or Equal?(x=w168, y=w169) -> (x >= y?=w166:bool)
          n79 = Or(x=w166, y=w161) -> (x .or. y?=w167:bool)
        }
        n80 = Increment(x=w153) -> (x+1=w152:i32)
        n81 = Array Size(array=w159) -> (size(s)=w157:i32)
      }
    }
  }
  "以各排數量切割之主要陣列" <- w2
  "各排數量" <- w13
  "處理點數y" <- w8
  n82 = Array Size(array=w13) -> (size(s)=w15:i32)
  n83 = for {
    N: w15 -> [_]
    tunnel: w13 -> [w179] mode=indexing
    tunnel: [w177] -> w14 mode=indexing
    shift-right: [w178] -> _
    shift-left: w12 -> [w180]
    n84 = Split 1D Array(array=w180, index=w179) -> (first subarray=w177:dbl[], second subarray=w178:dbl[])
  }
  "以各排數量切割之次要陣列" <- w14
  n85 = for {
    tunnel: w2 -> [w182] mode=indexing
    tunnel: w14 -> [w183] mode=indexing
    tunnel: [w184] -> w11 mode=indexing
    tunnel: "主排序參考目標" -> [w181]
    n86 = Build Cluster Array ("Index & Bundle Cluster Array")(w183, w182) -> (w186:cluster{"Y":dbl, "Y":dbl}[])
    n87 = Sort 1D Array(array=w186) -> (sorted array=w185:cluster{"Y":dbl, "Y":dbl}[])
    n88 = for {
      tunnel: w185 -> [w189] mode=indexing
      tunnel: [w190] -> w184 mode=indexing
      tunnel: w181 -> [w187]
      n89 = case shown="\"Y排序\", Default" w187 {
        tunnel: w189 -> [w191 w195]
        tunnel: [w191 w192] -> w188
        frame "Y排序", Default {
        }
        frame "X排序" {
          n90 = Unbundle(w195) -> ("Y"=w194:dbl, "Y"=w193:dbl)
          n91 = Bundle("Y"=w193, "Y"=w194) -> (w192:cluster{"Y":dbl, "Y":dbl})  [unwired: 1 in]
        }
      }
      n92 = Cluster To Array(cluster=w188) -> (array=w190:dbl[])
    }
  }
  "已完成排序陣列" <- w11
  n93 = for {
    tunnel: w11 -> [w197] mode=indexing
    tunnel: [w196] -> w10 mode=indexing
    n94 = for {
      tunnel: w197 -> [w202] mode=indexing
      tunnel: [w199] -> w196 mode=indexing
      n95 = Index Array(array=w202) -> (element #1=w201:dbl, element #2=w200:dbl)  [unwired: 2 in]
      n96 = Bundle(cluster=cluster{"X":dbl, "Y":dbl} {"X"=0.0, "Y"=0.0}, "X"=w201, "Y"=w200) -> (w199:cluster{"X":dbl, "Y":dbl})
    }
  }
  "已完成排序座標陣列" <- w10
  n97 = case shown="True" "繪出結果?" {
    tunnel: w10 -> [_ w203]
    frame False {
    }
    frame True {
      n98 = call "IMAQ Create"("Image Name"="1000") -> ("New Image"=w210:T1)  [unwired: 4 in, 1 out]
      n99 = call "IMAQ SetImageSize"("Y Resolution"=4500, "X Resolution"=11000 ("Y Resolution"), "Image"=w210) -> ("Image Out"=w204:T1)  [unwired: 2 in, 1 out]
      n100 = for {
        shift-right: [w213] -> _
        shift-left: w204 -> [w211]
        tunnel: errorcluster {"status"=FALSE, "code"=0, "source"=""} ("error constant") -> [w215]
        tunnel: [w214] -> w207 mode=indexing
        tunnel: w203 -> [w212] mode=indexing
        n101 = for {
          shift-right: [w216] -> w213
          shift-left: w211 -> [w223]
          shift-right: [w221] -> w214
          shift-left: w215 -> [w222]
          tunnel: w212 -> [w218] mode=indexing
          n102 = Build Array(w218) -> (w217:cluster{"X":dbl, "Y":dbl}[])
          n103 = Wait (ms)(milliseconds to wait=u32 0) -> ()  [unwired: 1 out]
          n104 = call "Overlay Points with User Specified Size.vi"("error in"=w222, "Point Diameter (5)"=u32 100, "Points"=w217, "Image In"=w223) -> ("error out"=w221:errorcluster, "Image Out"=w216:T1)  [unwired: 6 in]
          "Image" <- w216
        }
      }
      "Array 2" <- w207
    }
  }
